vi "Reanimate.vi"(8 "Error In":errorcluster, 11 "Selection List[]":refnum<vi>[](array[refnum])) -> (0 "Error Out":errorcluster, 3 "Change Made?":bool)   [LabVIEW 2017, in "Toolkit VIs.lvlib"]
doc: "Creates zombie code because once dead code is now alive (undead). Changes a grave site (Diagram Disable structure) to the Corpse frame (legacy code) and enables it. The \"Corpse\" label is replaced with a \"Zombie\" label and a timestamp of when the legacy code was re-enabled. In other words, infect the corpse with a zombie virus to revive it."
uses:
  Toolkit VIs.lvlib
  Typedefs/Bookmark Tags.ctl
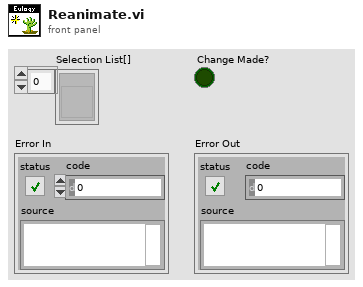
[diagram p1: front panel]
types:
  T1 = typedef "Toolkit VIs.lvlib/Bookmark Tags.ctl" = enum16{"RIP", "Zombie"}
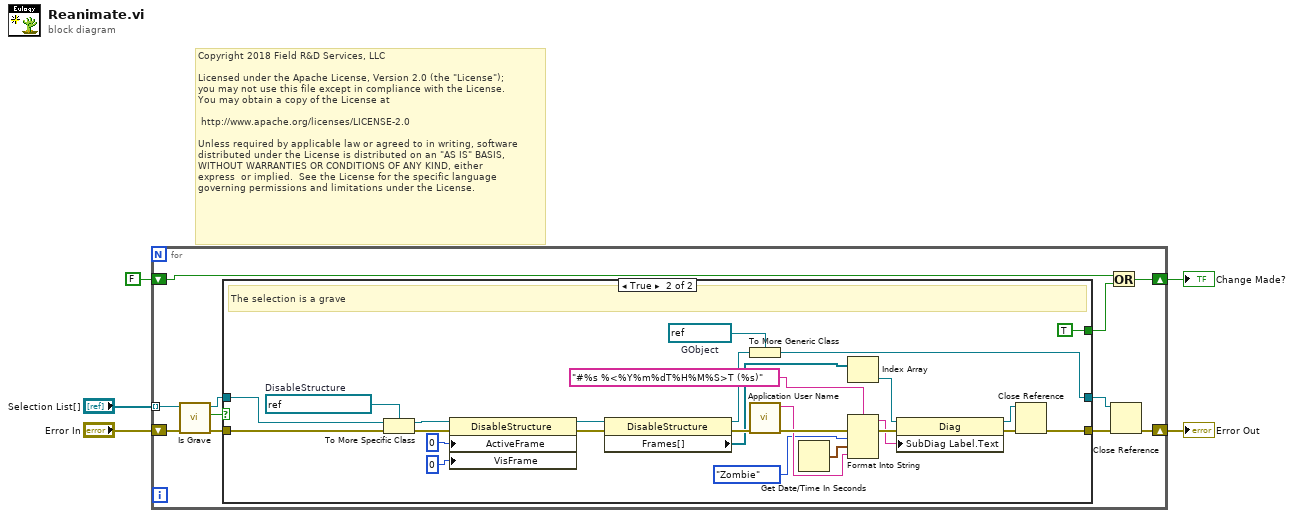
[diagram p0: block diagram]
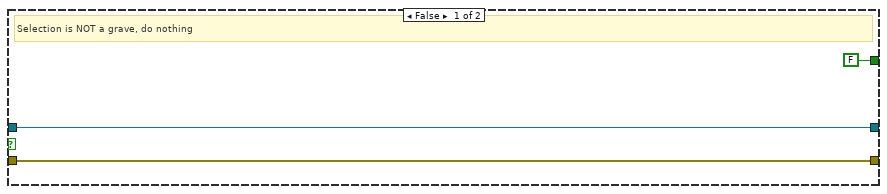
[diagram p2: hidden frame]
diagram:
  # "Copyright 2018 Field R&D Services, LLC\n\nLicensed under the Apache License, Version 2.0 (the \"License\");\nyou may not use this file except in compliance with the License.\nYou may obtain a copy of the License at\n\n\thttp://www.apache.org/licenses/LICENSE-2.0\n\nUnless required by applicable law or agreed to in writing, software\ndistributed under the License is distributed on an \"AS IS\" BASIS,\nWITHOUT WARRANTIES OR CONDITIONS OF ANY KIND, either \nexpress  or implied.  See the License for the specific language \ngoverning permissions and limitations under the License."
  n1 = for {
    shift-right: [w11] -> w5
    shift-left: "Error In" -> [w6]
    tunnel: "Selection List[]" -> [w10] mode=indexing
    shift-right: [w14] -> w3
    shift-left: FALSE -> [w16]
    n2 = call "Is Grave.vi"("Error In"=w6, "GObject In"=w10) -> ("Error Out"=w8:errorcluster, "Grave?"=w9:bool, "GObject Out"=w7:refnum<vi>)  [unwired: 7 in]
    n3 = case shown="True" w9 {
      tunnel: w8 -> [w18 w44]
      tunnel: [FALSE ("y") TRUE ("y")] -> w15
      tunnel: [w18 w42] -> w13
      tunnel: [w17 w40] -> w12
      tunnel: w7 -> [w17 w23]
      frame False {
        # "Selection is NOT a grave, do nothing"
      }
      frame True {
        w39 = refnum<vi> refnum  # GObject
        w45 = refnum<vi> refnum  # DisableStructure
        # "The selection is a grave"
        n4 = To More Specific Class(target class=w45, reference=w23, error in=w44) -> (specific class reference=w26:refnum<vi>, error out=w27:errorcluster)
        n5 = property class="DisableStructure"(reference=w26, error in=w27, "ActiveFrame"=i16 0 ("Active Frame"), "VisFrame"=u32 0 ("Visible Frame")) -> (reference out=w38:refnum<vi>, error out=w37:errorcluster)
        n6 = property class="DisableStructure"(reference=w38, error in=w37) -> (reference out=w41:refnum<vi>, error out=w33:errorcluster, "Frames[]"=w22:refnum<vi>[])
        n7 = To More Generic Class(target class=w39, reference=w41) -> (generic class reference=w40:refnum<vi>)
        n8 = call "Application User Name.vi"("Error In"=w33) -> ("Error Out"=w32:errorcluster, "User Name"=w29:string)  [unwired: 9 in]
        n9 = Get Date/Time In Seconds() -> (seconds since 1Jan1904=w30:timestamp)
        n10 = Index Array(array=w22) -> (element=w21:refnum<vi>)  [unwired: 1 in]
        n11 = Format Into String(format string="#%s %<%Y%m%dT%H%M%S>T (%s)" ("time format string (%c)"), error in=w32, Bookmark_Tags."Zombie" ("Bookmark"), w30, w29) -> (resulting string=w31:string, error out=w35:errorcluster)  [unwired: 1 in]
        n12 = property class="Diag"(reference=w21, error in=w35, "SubDiag Label.Text"=w31) -> (reference out=w20:refnum<vi>, error out=w36:errorcluster)
        n13 = Close Reference(reference=w20, error in (no error)=w36) -> (error out=w42:errorcluster)
      }
    }
    n14 = Or(x=w16, y=w15) -> (x .or. y?=w14:bool)
    n15 = Close Reference(reference=w12, error in (no error)=w13) -> (error out=w11:errorcluster)
  }
  "Error Out" <- w5
  "Change Made?" <- w3
